vi "CRYUpdate Insert Jump Info.vi"(7 "Jump State In":T1(array[cluster]), 8 "Count":i32, 9 "Steps In":T2[](array[typedef]) {"Repeat State Array"."Start" format="%#_5g"; "Y dB ref" format="%.1f"; "Y data" items=["dB", "Lin"]; "Start" format="%#_5g"}, 10 "Step number Selected":i32, 11 "Action":T3(ring)) -> (1 "Steps Out":T2[](array[typedef]) {"Repeat State Array"."Start" format="%#_5g"; "Y dB ref" format="%.1f"; "Y data" items=["dB", "Lin"]; "Start" format="%#_5g"}, 2 "Canceled?":bool)   [LabVIEW 2013]
uses:
  CRYSystem/Typedef Control/CRYStep.ctl
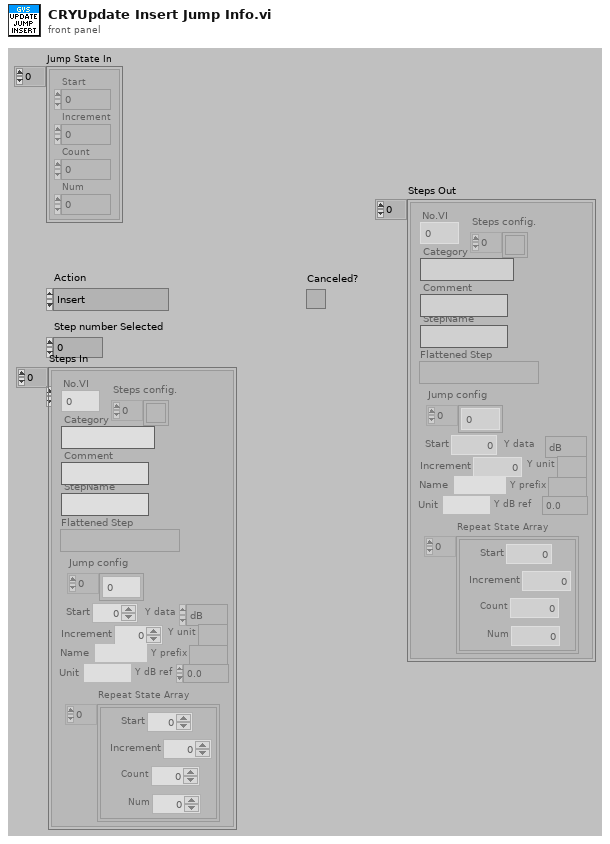
[diagram p1: front panel]
types:
  T1 = cluster{"Start":dbl, "Increment":dbl, "Count":i32, "Num":i32}[]
  T2 = typedef "CRYStep.ctl" = cluster{"No.VI":i32, "Category":string, "StepName":string, "Seq setup flattened":string, "Comment":string, "Steps config.":bool[], "Jump config":i32[], "Start":dbl, "Increment":dbl, "Name":string, "Unit":string, "Y data":u16, "Y prefix":string, "Y dB ref":dbl, "Y unit":string, "Repeat State Array":cluster{"Start":dbl, "Increment":dbl, "Count":i32, "Num":i32}[]}
  T3 = enum16{"Insert", "Remove", "Move up", "Move down"}
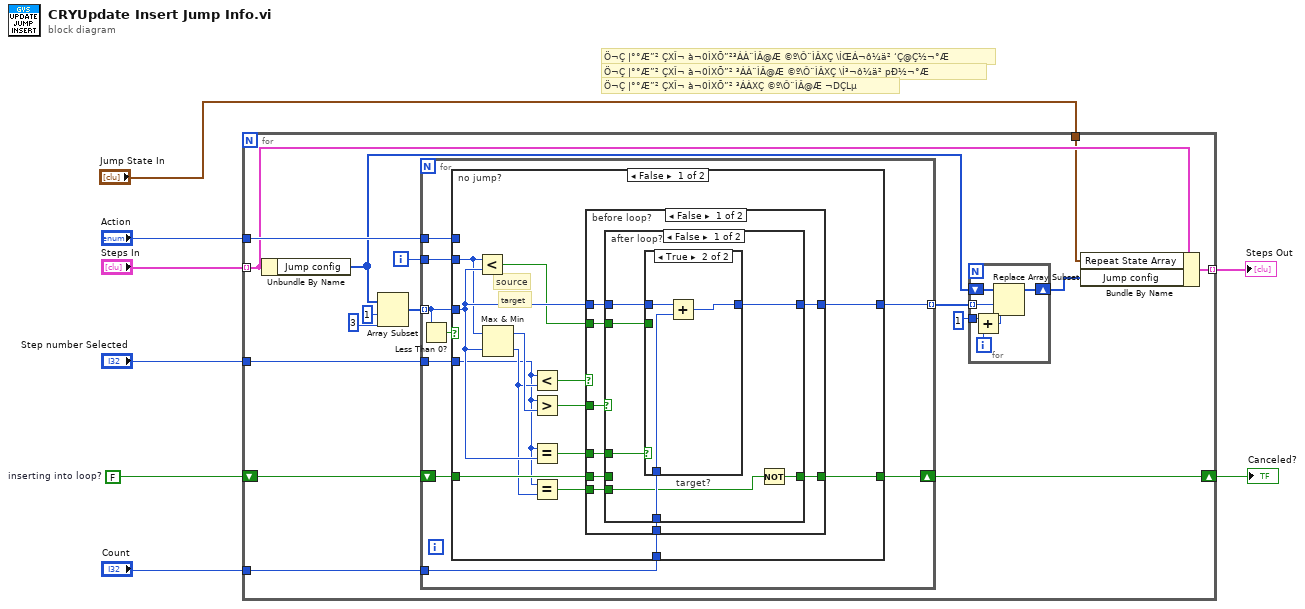
[diagram p0: block diagram]
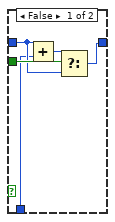
[diagram p2: hidden frame]
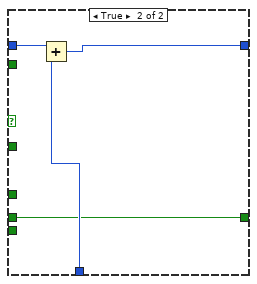
[diagram p4: hidden frame]
diagram:
  w5 = FALSE  # inserting into loop?
  # "Ö¬Ç |°°Æ”² ÇXÎ¬ à¬0ÌXÕ”² ³ÁÀXÇ ©º\\Ô¨ÌÂ@Æ ¬DÇLµ"
  # "Ö¬Ç |°°Æ”² ÇXÎ¬ à¬0ÌXÕ”² ³ÁÀ¨ÌÂ@Æ ©º\\Ô¨ÌÂXÇ \\Í³¬ô¼ä² pÐ½¬°Æ"
  # "Ö¬Ç |°°Æ”² ÇXÎ¬ à¬0ÌXÕ”²³ÁÀ¨ÌÂ@Æ ©º\\Ô¨ÌÂXÇ \\ÍŒÁ¬ô¼ä² ‘Ç@Ç½¬°Æ"
  n1 = for {
    tunnel: "Step number Selected" -> [w21]
    tunnel: "Action" -> [w20]
    tunnel: "Count" -> [w17]
    shift-right: [w15] -> w2
    shift-left: w5 -> [w16]
    tunnel: "Steps In" -> [w12] mode=indexing
    tunnel: [w11] -> w3 mode=indexing
    tunnel: "Jump State In" -> [w9]
    i -> [w22]
    n2 = Unbundle By Name(w12) -> ("Jump config"=w13:i32[])
    n3 = Array Subset(array=w13, index=1, length=3) -> (w14:i32[])
    n4 = for {
      tunnel: w14 -> [w38] mode=indexing
      tunnel: w22 -> [w37]
      tunnel: w21 -> [w36]
      tunnel: w20 -> [w35]
      tunnel: [w34] -> w18 mode=indexing
      tunnel: w17 -> [w33]
      shift-right: [w32] -> w15
      shift-left: w16 -> [w31]
      n5 = Less Than 0?(x=w38) -> (x < 0?=w39:bool)
      n6 = case "no jump?" shown="False" w39 {
        tunnel: w38 -> [w49 w85]
        tunnel: w37 -> [w46 _]
        tunnel: w36 -> [w41 _]
        tunnel: w35 -> [_ _]
        tunnel: [w52 w85] -> w34
        tunnel: w33 -> [w45 _]
        tunnel: [w44 w84] -> w32
        tunnel: w31 -> [w43 w84]
        frame False {
          # "target"
          # "source"
          n7 = Less?(x=w46, y=w49) -> (x < y?=w47:bool)
          n8 = Max & Min(x=w46, y=w49) -> (max(x,y)=w50:i32, min(x,y)=w42:i32)
          n9 = Less?(x=w41, y=w42) -> (x < y?=w53:bool)
          n10 = Greater?(x=w41, y=w50) -> (0:w51:bool)
          n11 = Equal?(x=w41, y=w49) -> (x = y?=w48:bool)
          n12 = Equal?(x=w41, y=w42) -> (x = y?=w40:bool)
          n13 = case "before loop?" shown="False" w53 {
            tunnel: w49 -> [w61 w83]
            tunnel: [w60 w81] -> w52
            tunnel: w51 -> [w62 _]
            tunnel: w48 -> [w59 _]
            tunnel: w47 -> [w58 _]
            tunnel: w45 -> [w57 w82]
            tunnel: [w56 w80] -> w44
            tunnel: w43 -> [w55 w80]
            tunnel: w40 -> [w54 _]
            frame False {
              n14 = case "after loop?" shown="False" w62 {
                tunnel: [w68 w79] -> w60
                tunnel: w61 -> [w67 w79]
                tunnel: w59 -> [w69 _]
                tunnel: w58 -> [w66 _]
                tunnel: w57 -> [w65 _]
                tunnel: [w63 w78] -> w56
                tunnel: w55 -> [_ w78]
                tunnel: w54 -> [w64 _]
                frame False {
                  n15 = case "target?" shown="True" w69 {
                    tunnel: [w74 w76] -> w68
                    tunnel: w67 -> [w72 w77]
                    tunnel: w66 -> [w73 _]
                    tunnel: w65 -> [w70 w75]
                    frame False {
                      n16 = Add(x=w72, y=w70) -> (x+y=w71:i32)
                      n17 = Select(t=w71, s=w73, f=w72) -> (s? t:f=w74:i32)
                    }
                    frame True {
                      n18 = Add(x=w77, y=w75) -> (x+y=w76:i32)
                    }
                  }
                  n19 = Not(x=w64) -> (.not. x?=w63:bool)
                }
                frame True {
                }
              }
            }
            frame True {
              n20 = Add(x=w83, y=w82) -> (x+y=w81:i32)
            }
          }
        }
        frame True {
        }
      }
    }
    n21 = for {
      tunnel: 1 -> [w28]
      tunnel: w18 -> [w27] mode=indexing
      shift-right: [w25] -> w10
      shift-left: w13 -> [w26]
      i -> [w30]
      n22 = Add(x=w28, y=w30) -> (x+y=w29:i32)
      n23 = Replace Array Subset(array=w26, new element=w27, index=w29) -> (w25:i32[])
    }
    n24 = Bundle By Name(cluster=w12, "Repeat State Array"=w9, "Jump config"=w10) -> (w11:T2)
  }
  "Canceled?" <- w2
  "Steps Out" <- w3
